vi "roboRIO v1.0 Get Scaling Constants.vi"(8 "error in (no error)":errorcluster, 11 "Channel Name":string) -> (0 "error out":errorcluster, 3 "Channel Scaling":u32[](array[numeric]))   [LabVIEW 2021]
uses:
  <vilib>/myRIO/Common/Instrument Driver Framework/roboRIO v1.0/Resource Manager/vis/roboRIO v1.0 Scaling Constants Table.vi
  <vilib>/Utility/error.llb/Trim Whitespace.vi
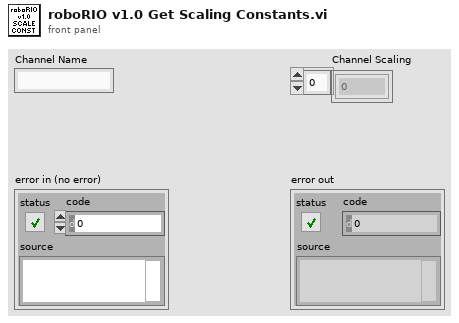
[diagram p1: front panel]
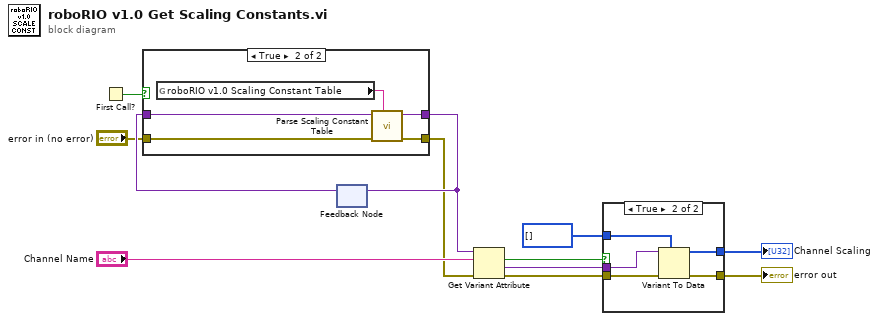
[diagram p0: block diagram]
diagram:
  n1 = First Call?() -> (First Call?: T/F=w3:bool)
  n2 = feedback #1() -> (w4:variant)  [unwired: 1 in]
  n3 = case shown="True" w3 {
    tunnel: [w14 w17] -> w5
    tunnel: w4 -> [w14 w18]
    tunnel: "error in (no error)" -> [w13 w15]
    tunnel: [w13 w16] -> w1
    frame False {
    }
    frame True {
      n4 = global read "roboRIO v1.0 Scaling Constants Table.vi" "roboRIO v1.0 Scaling Constant Table"() -> (w19:string)
      n5 = call <vilib>:"Parse Scaling Constant Table.vi"("Scaling Constant Table"=w19, "error in (no error)"=w15, "Variant in"=w18) -> ("error out"=w16:errorcluster, "Variant out"=w17:variant)  [unwired: 7 in]
    }
  }
  n6 = feedback-in #1(w5) -> ()
  n7 = Get Variant Attribute(Variant=w5, name="Channel Name", error in=w1) -> (found=w8:bool, value=w9:variant, error out=w7:errorcluster)  [unwired: 1 in, 1 out]
  n8 = case shown="True" w8 {
    tunnel: u32[] [] ("Channel Scaling") -> [w21 w26]
    tunnel: [w21 w25] -> w10
    tunnel: w9 -> [_ w24]
    tunnel: w7 -> [w20 w23]
    tunnel: [w20 w22] -> w6
    frame False {
    }
    frame True {
      n9 = Variant To Data(error in=w23, type=w26, Variant=w24) -> (data=w25:u32[], error out=w22:errorcluster)
    }
  }
  "error out" <- w6
  "Channel Scaling" <- w10
